vi "ma_sml_Compensation Filter Design.vi"(2 "stop band attenuation":enum16{"84 dB", "96 dB", "120 dB"}(ring)=enum."120 dB", 3 "M":i32=256) -> (0 "CIC stages":i32=7, 1 "filter coefficients":dbl[](graph))   [LabVIEW 2020, in "NI_MAPro.lvlib"]
uses:
  NI_MAPro.lvlib
  NI_AALBase.lvlib
  NI_AALPro.lvlib
panel:
  in  "debug?":bool
  in  "WEIGHT":dbl=10.0 format="%.2f"
  out "pass band error":dbl[](graph)
  in  "#of compensation points":i32=30
  in  "linear/log":bool
  out "frequency response":cluster{"Element Data":dbl, dbl, dbl[]}(graph)={"Element Data"=0.0, 1.52587890625e-05, []}
  out "error":i32
  out "ripple":dbl=1.1396470425114667e-06 format="%.2e"
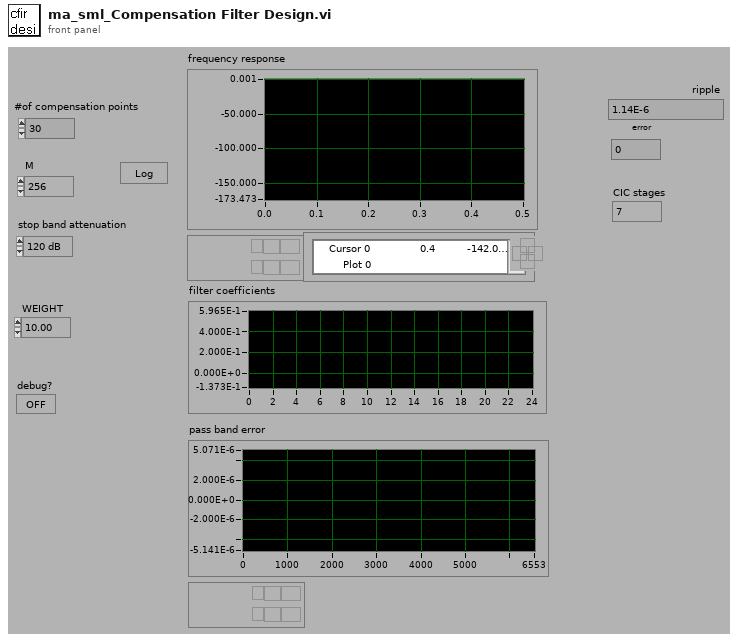
[diagram p1: front panel]
types:
  T1 = cluster{"Element Data":dbl, "Element Data":dbl, "Element Data":dbl, "WEIGHT":dbl}[]
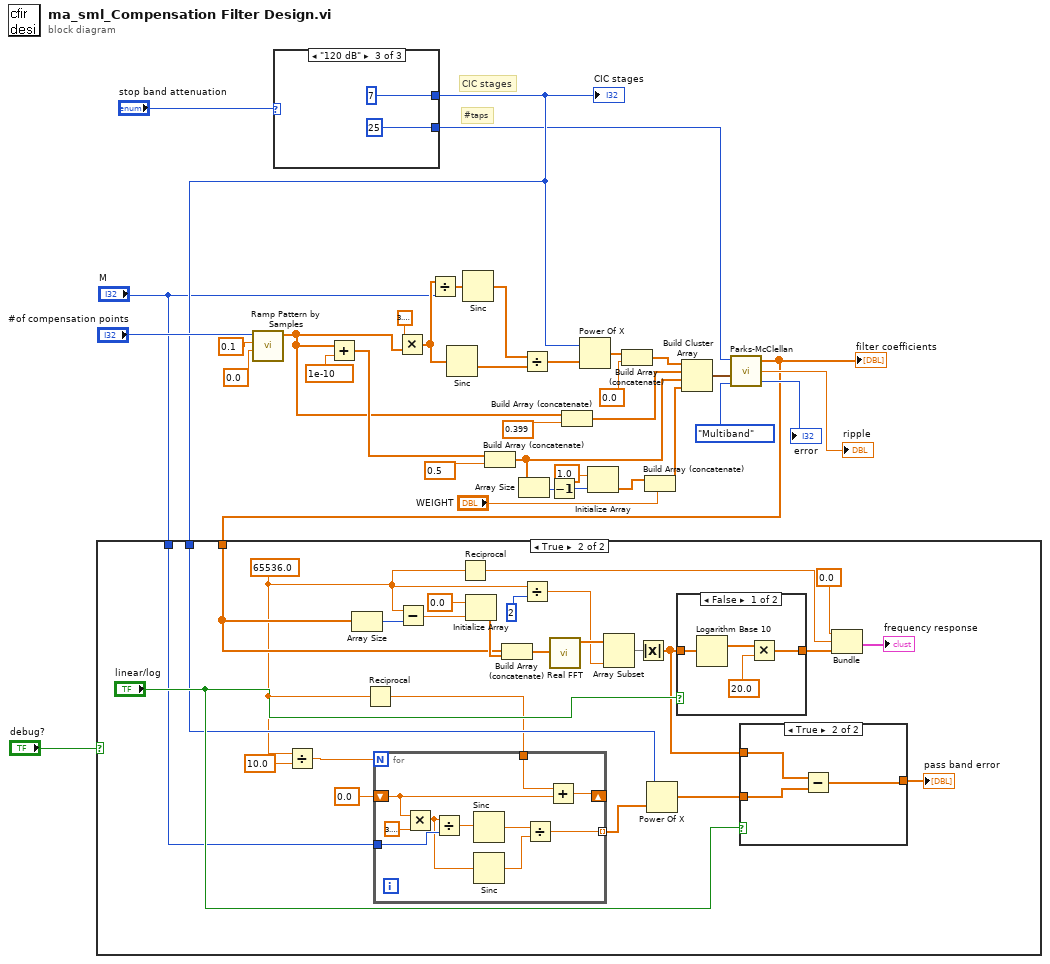
[diagram p0: block diagram]
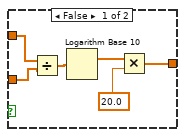
[diagram p3: hidden frame]
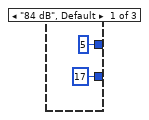
[diagram p5: hidden frame]
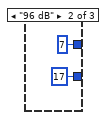
[diagram p6: hidden frame]
diagram:
  # "#taps"
  # "CIC stages"
  n1 = call "Ramp Pattern by Samples.vi"("start"=0.0, "end"=0.1, "samples"="#of compensation points") -> ("Ramp Pattern"=w9:dbl[])  [unwired: 7 in, 1 out]
  n2 = case shown="\"120 dB\"" "stop band attenuation" {
    tunnel: [5 7 7] -> w13
    tunnel: [17 17 25] -> w12
    frame "84 dB", Default {
    }
    frame "96 dB" {
    }
    frame "120 dB" {
    }
  }
  "CIC stages" <- w13
  n3 = Add(x=w9, y=1e-10 ("Element Data")) -> (x+y=w23:dbl[])
  n4 = Multiply(x=3.141592653589793, y=w9) -> (x*y=w10:dbl[])
  n5 = Divide(x=w10, y="M") -> (x/y=w11:dbl[])
  n6 = Sinc(1:w10) -> (0:w7:dbl[])
  n7 = Sinc(1:w11) -> (0:w8:dbl[])
  n8 = Build Array (concatenate)(w23, 0.5 ("Element Data")) -> (w19:dbl[])
  n9 = Array Size(array=w19) -> (size(s)=w30:i32)
  n10 = Divide(x=w8, y=w7) -> (x/y=w6:dbl[])
  n11 = Decrement(x=w30) -> (x-1=w5:i32)
  n12 = Build Array (concatenate)(w9, 0.399 ("Element Data")) -> (w24:dbl[])
  n13 = Power Of X(1:w6, 2:w13) -> (0:w20:dbl[])
  n14 = Initialize Array(1.0 ("Element Data"), w5) -> (w28:dbl[])
  n15 = Build Array (concatenate)(w20, 0.0 ("Element Data")) -> (w32:dbl[])
  n16 = Build Array (concatenate)(w28, "WEIGHT") -> (w4:dbl[])
  n17 = Build Cluster Array(w32, w24, w19, w4) -> (w25:T1)
  n18 = call "Parks-McClellan.vi"("filter type"=enum32{"Multiband", "Differentiator", "Hilbert"}."Multiband", "Band Parameters"=w25, "# of taps"=w12) -> ("error"=→"error":i32, "ripple"=→"ripple":dbl, "h"=w15:dbl[])  [unwired: 1 in]
  "filter coefficients" <- w15
  n19 = case shown="True" "debug?" {
    tunnel: w15 -> [_ w50]
    tunnel: w13 -> [_ w49]
    tunnel: "M" -> [_ w42]
    frame False {
    }
    frame True {
      w47 = 65536.0 ("Element Data")
      n20 = Divide(x=w47, y=10.0) -> (x/y=w48:dbl)
      n21 = Array Size(array=w50) -> (size(s)=w64:i32)
      n22 = Reciprocal(x=w47) -> (1/x=w43:dbl)
      n23 = for {
        N: w48 -> [_]
        shift-right: [w69] -> _
        shift-left: 0.0 -> [w70]
        tunnel: w42 -> [w76]
        tunnel: [w71] -> w44 mode=indexing
        tunnel: w43 -> [w68]
        n24 = Multiply(x=w70, y=3.141592653589793) -> (x*y=w74:dbl)
        n25 = Divide(x=w74, y=w76) -> (x/y=w75:dbl)
        n26 = Sinc(1:w75) -> (0:w73:dbl)
        n27 = Sinc(1:w74) -> (0:w72:dbl)
        n28 = Divide(x=w73, y=w72) -> (x/y=w71:dbl)
        n29 = Add(x=w68, y=w70) -> (x+y=w69:dbl)
      }
      n30 = Subtract(x=w47, y=w64) -> (x-y=w59:dbl)
      n31 = Reciprocal(x=w47) -> (1/x=w55:dbl)
      n32 = Initialize Array(0.0 ("Element Data"), w59) -> (w66:dbl[])
      n33 = Build Array (concatenate)(w50, w66) -> (w58:dbl[])
      n34 = Divide(x=w47, y=2) -> (x/y=w62:dbl)
      n35 = call "Real FFT.vi"("X"=w58) -> ("FFT {X}"=w65:cdb[])  [unwired: 9 in, 1 out]
      n36 = Array Subset(array=w65, length=w62) -> (w61:cdb[])  [unwired: 1 in]
      n37 = Absolute Value(x=w61) -> (abs(x)=w51:dbl[])
      n38 = Power Of X(1:w44, 2:w49) -> (0:w52:dbl[])
      n39 = case shown="False" "linear/log" {
        tunnel: w51 -> [w90 w91]
        tunnel: [w89 w91] -> w56
        frame False {
          n40 = Logarithm Base 10(1:w90) -> (0:w88:dbl[])
          n41 = Multiply(x=w88, y=20.0 ("Element Data")) -> (x*y=w89:dbl[])
        }
        frame True {
        }
      }
      n42 = case shown="True" "linear/log" {
        tunnel: [w83 w84] -> w53
        tunnel: w51 -> [w79 w86]
        tunnel: w52 -> [w78 w85]
        frame False {
          n43 = Divide(x=w79, y=w78) -> (x/y=w80:dbl[])
          n44 = Logarithm Base 10(1:w80) -> (0:w82:dbl[])
          n45 = Multiply(x=w82, y=20.0 ("Element Data")) -> (x*y=w83:dbl[])
        }
        frame True {
          n46 = Subtract(x=w86, y=w85) -> (x-y=w84:dbl[])
        }
      }
      "pass band error" <- w53
      n47 = Bundle("Element Data"=0.0, w55, w56) -> (→"frequency response":cluster{"Element Data":dbl, dbl, dbl[]})  [unwired: 1 out]
    }
  }
